vi "START EDIT SETTINGS.vi"(11 "REFERENCES":T1) -> ()   [LabVIEW 2019]
uses:
  Controls/References Cluster.ctl
  <vilib>/userDefined/High Color/IMAQdx.ctl
  Controls/Custom Calendar/Custom Calendar.xctl
  <vilib>/Utility/miscctls.llb/LVRowAndColumnTypeDef.ctl
  <vilib>/addons/database/Connection.llb/DB Tools Open Connec (String).vi
  <vilib>/addons/database/_DB Variant To Data/Database Variant To Data.xnode
  <vilib>/addons/database/NI_Database_API.lvlib
types:
  T1 = typedef "References Cluster.ctl" = cluster{"MAIN PAGES":refnum<vi>, "ADD/EDIT ITEM REFERENCES":cluster{"Identifier":refnum<vi>, "BYU ICN #":refnum<vi>, "Item Description":refnum<vi>, "Comments":refnum<vi>, "Checked Out Date":refnum<vi>, "Due Date":refnum<vi>, "Check Out Location":refnum<vi>, "Reminder Count":refnum<vi>, "Most Recent Reminder Date":refnum<vi>, "BYU ID #":refnum<vi>, "Building/Room":refnum<vi>, "Location in Room":refnum<vi>, "Manual":refnum<vi>, "Manufacturer":refnum<vi>, "Model #":refnum<vi>, "Serial #":refnum<vi>, "Date Acquired":refnum<vi>, "ADD/EDIT ITEM LABEL":refnum<vi>, "ARCHIVE ITEM":refnum<vi>, "Archive Item Inputs":refnum<vi>, "Reminder Notes":refnum<vi>, "DUPLICATE ITEM":refnum<vi>}, "ADD/EDIT USER REFERENCES":cluster{"BYU ID # (##-###-####)":refnum<vi>, "First Name":refnum<vi>, "Last Name":refnum<vi>, "Phone Number (###-###-####)":refnum<vi>, "Email":refnum<vi>, "Department":refnum<vi>, "Graduation Status":refnum<vi>, "Anticipated Graduation Year":refnum<vi>, "Credit Score":refnum<vi>, "Date Added":refnum<vi>, "Graduation Clearance Date":refnum<vi>, "Picture File Name":refnum<vi>, "ADD/EDIT USER LABEL":refnum<vi>, "Department Map":refnum<vi>, "Status Map":refnum<vi>, "Anticipated Graduation Year Map":refnum<vi>, "User Agreement":refnum<vi>, "User Comments":refnum<vi>, "Camera":refnum<vi>}, "RETURN ITEM REFERENCES":cluster{"Item or Person:":refnum<vi>, "Search Return Results":refnum<vi>, "What are you searching for?":refnum<vi>}, "SEARCH DATABASE REFERENCES":cluster{"What to Search For:":refnum<vi>, "Where to Search":refnum<vi>, "Column to Search In":refnum<vi>, "Column to Sort By":refnum<vi>, "Search Database Results":refnum<vi>, "Inventory Column Selector":refnum<vi>, "User Column Selector":refnum<vi>, "Inventory Archive Column Selector":refnum<vi>, "User Archive Column Selector":refnum<vi>, "Sales Tracking Column Selector":refnum<vi>, "Checked In Archive Column Selector":refnum<vi>, "Restore User":refnum<vi>, "Date Range":refnum<vi>, "Dates Less Than":refnum<vi>, "Dates Greater Than":refnum<vi>, "Search Print Receipt":refnum<vi>, "Edit Sale Description":refnum<vi>}, "USER ITEMS REFERENCES":cluster{"USER'S INFORMATION":refnum<vi>, "User's Checked Out Items":refnum<vi>, "User Info Comments":refnum<vi>, "SEE USER INFO COMMENTS":refnum<vi>}, "EDIT ITEMS REFERENCES":cluster{"New Check Out Location":refnum<vi>, "Items to Edit":refnum<vi>, "Edit Items Due Date":refnum<vi>, "New Reminder Notes":refnum<vi>, "New Item Description":refnum<vi>}, "CHECK OUT ITEMS REFERENCES":cluster{"Enter Item:":refnum<vi>, "Check Out Items Due Date":refnum<vi>, "Check Out Location":refnum<vi>, "Items to be Checked Out":refnum<vi>, "Possible Items":refnum<vi>, "Altered Item Description":refnum<vi>}, "TRANSFER ITEMS REFERENCES":cluster{"Search Parameter":refnum<vi>, "What to Match":refnum<vi>, "Matching Individuals":refnum<vi>, "Items to be Transferred":refnum<vi>}, "SETTINGS REFERENCES":cluster{"PSC Database Settings":refnum<vi>, "PSC Sales Item Spreadsheet":refnum<vi>}, "PSC SALES REFERENCES":cluster{"BYU ID CARD #":refnum<vi>, "Sale Description":refnum<vi>, "Scan or Enter Item Name":refnum<vi>, "Items to be Sold":refnum<vi>, "Grand Total":refnum<vi>, "Item List":refnum<vi>}}
  T2 = typedef "LVRowAndColumnTypeDef.ctl" = cluster{"Row":i32, "Column":i32}
  T3 = typedef "NI_Database_API.lvlib/Conn ObjectReference.ctl" = refnum<k1>
  T4 = cluster{"PSC Database Settings":refnum<vi>, "PSC Sales Item Spreadsheet":refnum<vi>}
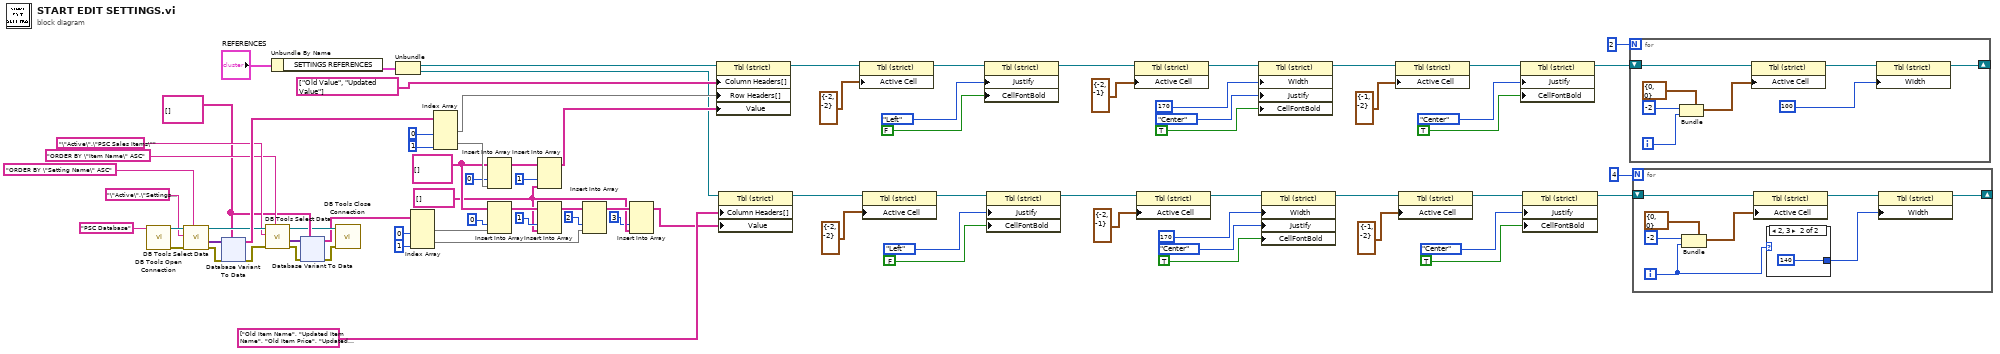
[diagram p0: block diagram]
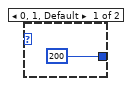
[diagram p2: hidden frame]
diagram:
  w3 = string[] []
  w12 = string[][] []
  w19 = string[][] []
  n1 = call-poly <vilib>:"DB Tools Open Connection.vi"("connection information"="PSC Database") -> ("error out"=w79:errorcluster, "connection reference"=w78:T3)  [unwired: 7 in]
  n2 = call <vilib>:"DB Tools Select Data.vi"("condition"="ORDER BY \"Setting Name\" ASC", "error in (no error)"=w79, "table"="\"Active\".\"Settings\"", "connection reference"=w78) -> ("error out"=w76:errorcluster, "data"=w75:variant[][], "connection reference out"=w25:T3)  [unwired: 2 in]
  n3 = xnode "Database Variant To Data"("database variant"=w75, "error in (no error)"=w76, "type"=w19) -> ("data"=w74:string[][], "error out"=w22:errorcluster)
  n4 = call <vilib>:"DB Tools Select Data.vi"("condition"="ORDER BY \"Item Name\" ASC", "error in (no error)"=w22, "table"="\"Active\".\"PSC Sales Items\"", "connection reference"=w25) -> ("error out"=w20:errorcluster, "data"=w21:variant[][], "connection reference out"=w18:T3)  [unwired: 2 in]
  n5 = Unbundle By Name("REFERENCES") -> ("SETTINGS REFERENCES"=w81:T4)
  n6 = xnode "Database Variant To Data"("database variant"=w21, "error in (no error)"=w20, "type"=w19) -> ("data"=w15:string[][], "error out"=w17:errorcluster)
  n7 = call <vilib>:"DB Tools Close Connection.vi"("error in (no error)"=w17, "connection reference"=w18) -> ()  [unwired: 5 in, 1 out]
  n8 = Unbundle(w81) -> ("PSC Database Settings"=w72:refnum<vi>, "PSC Sales Item Spreadsheet"=w26:refnum<vi>)
  n9 = Index Array(array=w15, index (col) #1=0 ("disabled index (col)"), index (col) #2=1 ("index (col)")) -> (element #1=w9:string[], element #2=w5:string[])  [unwired: 2 in]
  n10 = Index Array(array=w74, index (col) #1=0 ("disabled index (col)"), index (col) #2=1 ("index (col)")) -> (element #1=w70:string[], element #2=w68:string[])  [unwired: 2 in]
  n11 = Insert Into Array(array=w12, index (col)=0 ("disabled index (col)"), new element=w68) -> (w66:string[][])  [unwired: 1 in]
  n12 = Insert Into Array(array=w12, index (col)=0 ("disabled index (col)"), new element=w9) -> (w10:string[][])  [unwired: 1 in]
  n13 = Insert Into Array(array=w66, index (col)=1 ("disabled index (col)"), new element=w3) -> (w64:string[][])  [unwired: 1 in]
  n14 = Insert Into Array(array=w10, index (col)=1 ("disabled index (col)"), new element=w3) -> (w7:string[][])  [unwired: 1 in]
  n15 = Insert Into Array(array=w7, index (col)=2 ("disabled index (col)"), new element=w5) -> (w4:string[][])  [unwired: 1 in]
  n16 = Insert Into Array(array=w4, index (col)=3 ("disabled index (col)"), new element=w3) -> (w1:string[][])  [unwired: 1 in]
  n17 = property class="Tbl (strict)"(reference=w72, "Column Headers[]"=string[] ["Old Value", "Updated Value"] ("Column Header Strings[]"), "Row Headers[]"=w70, "Value"=w64) -> (reference out=w49:refnum<vi>)  [unwired: 1 in, 1 out]
  n18 = property class="Tbl (strict)"(reference=w26, "Column Headers[]"=string[] ["Old Item Name", "Updated Item  Name", "Old Item Price", "Updated Item Price"] ("Column Header Strings[]"), "Value"=w1) -> (reference out=w41:refnum<vi>)  [unwired: 1 in, 1 out]
  n19 = property class="Tbl (strict)"(reference=w49, "Active Cell"=T2 {"Row"=-2, "Column"=-2} ("Active Cell:Active Cell")) -> (reference out=w52:refnum<vi>)  [unwired: 1 in, 1 out]
  n20 = property class="Tbl (strict)"(reference=w41, "Active Cell"=T2 {"Row"=-2, "Column"=-2} ("Active Cell:Active Cell")) -> (reference out=w38:refnum<vi>)  [unwired: 1 in, 1 out]
  n21 = property class="Tbl (strict)"(reference=w52, "Justify"=enum16{"Left", "Center", "Right"}."Left" ("Active Cell:Cell Justification"), "CellFontBold"=FALSE ("Active Cell:Cell Font:Bold")) -> (reference out=w48:refnum<vi>)  [unwired: 1 in, 1 out]
  n22 = property class="Tbl (strict)"(reference=w38, "Justify"=enum16{"Left", "Center", "Right"}."Left" ("Active Cell:Cell Justification"), "CellFontBold"=FALSE ("Active Cell:Cell Font:Bold")) -> (reference out=w42:refnum<vi>)  [unwired: 1 in, 1 out]
  n23 = property class="Tbl (strict)"(reference=w48, "Active Cell"=T2 {"Row"=-2, "Column"=-1} ("Active Cell:Active Cell")) -> (reference out=w62:refnum<vi>)  [unwired: 1 in, 1 out]
  n24 = property class="Tbl (strict)"(reference=w42, "Active Cell"=T2 {"Row"=-2, "Column"=-1} ("Active Cell:Active Cell")) -> (reference out=w28:refnum<vi>)  [unwired: 1 in, 1 out]
  n25 = property class="Tbl (strict)"(reference=w62, "Width"=u32 170 ("Active Cell:Cell Size:Width"), "Justify"=enum16{"Left", "Center", "Right"}."Center" ("Active Cell:Cell Justification"), "CellFontBold"=TRUE ("Active Cell:Cell Font:Bold")) -> (reference out=w54:refnum<vi>)  [unwired: 1 in, 1 out]
  n26 = property class="Tbl (strict)"(reference=w28, "Width"=u32 170 ("Active Cell:Cell Size:Width"), "Justify"=enum16{"Left", "Center", "Right"}."Center" ("Active Cell:Cell Justification"), "CellFontBold"=TRUE ("Active Cell:Cell Font:Bold")) -> (reference out=w36:refnum<vi>)  [unwired: 1 in, 1 out]
  n27 = property class="Tbl (strict)"(reference=w54, "Active Cell"=T2 {"Row"=-1, "Column"=-2} ("Active Cell:Active Cell")) -> (reference out=w56:refnum<vi>)  [unwired: 1 in, 1 out]
  n28 = property class="Tbl (strict)"(reference=w36, "Active Cell"=T2 {"Row"=-1, "Column"=-2} ("Active Cell:Active Cell")) -> (reference out=w34:refnum<vi>)  [unwired: 1 in, 1 out]
  n29 = property class="Tbl (strict)"(reference=w56, "Justify"=enum16{"Left", "Center", "Right"}."Center" ("Active Cell:Cell Justification"), "CellFontBold"=TRUE ("Active Cell:Cell Font:Bold")) -> (reference out=w47:refnum<vi>)  [unwired: 1 in, 1 out]
  n30 = property class="Tbl (strict)"(reference=w34, "Justify"=enum16{"Left", "Center", "Right"}."Center" ("Active Cell:Cell Justification"), "CellFontBold"=TRUE ("Active Cell:Cell Font:Bold")) -> (reference out=w43:refnum<vi>)  [unwired: 1 in, 1 out]
  n31 = for {
    N: 2 -> [_]
    shift-right: [w84] -> _
    shift-left: w47 -> [w85]
    i -> [w88]
    n32 = Bundle(cluster=T2 {"Row"=0, "Column"=0} ("Active Cell:Active Cell"), "Row"=-2, "Column"=w88) -> (w86:T2)
    n33 = property class="Tbl (strict)"(reference=w85, "Active Cell"=w86) -> (reference out=w90:refnum<vi>)  [unwired: 1 in, 1 out]
    n34 = property class="Tbl (strict)"(reference=w90, "Width"=u32 100 ("Active Cell:Cell Size:Width")) -> (reference out=w84:refnum<vi>)  [unwired: 1 in, 1 out]
  }
  n35 = for {
    N: 4 -> [_]
    shift-right: [w93] -> _
    shift-left: w43 -> [w94]
    i -> [w91]
    n36 = Bundle(cluster=T2 {"Row"=0, "Column"=0} ("Active Cell:Active Cell"), "Row"=-2, "Column"=w91) -> (w95:T2)
    n37 = property class="Tbl (strict)"(reference=w94, "Active Cell"=w95) -> (reference out=w98:refnum<vi>)  [unwired: 1 in, 1 out]
    n38 = case shown="2, 3" w91 {
      tunnel: [u32 200 ("Active Cell:Cell Size:Width") u32 140 ("Active Cell:Cell Size:Width")] -> w92
      frame 0, 1, Default {
      }
      frame 2, 3 {
      }
    }
    n39 = property class="Tbl (strict)"(reference=w98, "Width"=w92) -> (reference out=w93:refnum<vi>)  [unwired: 1 in, 1 out]
  }
